vi "getAllSpectraFromFolder.vi"(11 "Spectra Folder::":path) -> (2 "spectra":dbl[][][](array[numeric]) caption="spectrum\n\n\nFrequency\n\n\nColumn")   [LabVIEW 2013]
panel:
  out "All Spec Files in Dir":path[](array[path])
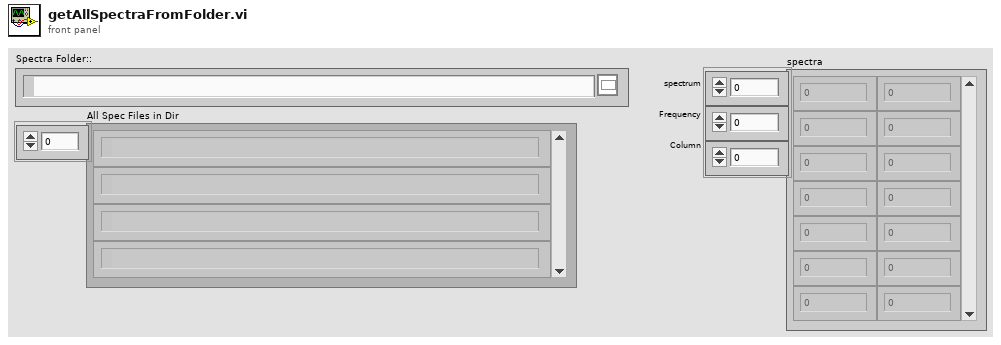
[diagram p1: front panel]
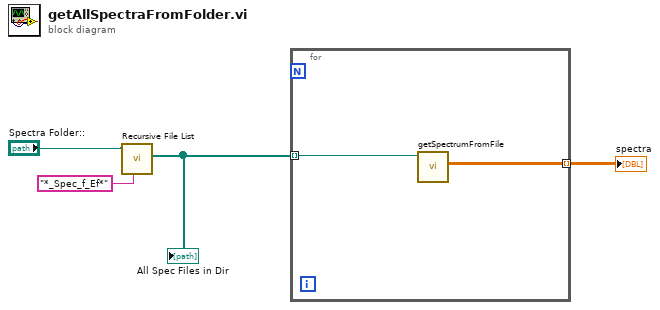
[diagram p0: block diagram]
diagram:
  n1 = call <vilib>:"Recursive File List.vi"("pattern"="*_Spec_f_Ef*", "Folder Path"="Spectra Folder::") -> ("All Files in Dir"=w3:path[])  [unwired: 5 in, 4 out]
  "All Spec Files in Dir" <- w3
  n2 = for {
    tunnel: w3 -> [w5] mode=indexing
    tunnel: [w6] -> w2 mode=indexing
    n3 = call "getSpectrumFromFile.vi"("File Path Control"=w5) -> ("array"=w6:dbl[][])  [unwired: 10 in]
  }
  "spectra" <- w2
